vi "3-1.vi"(9 "信号数组(V)":dbl[](array[numeric]), 10 "编码位数L":dbl=8.0, 11 "量化阶Δ(V)":dbl=0.02) -> (3 "还原信号数组(V)":dbl[](array[numeric]))   [LabVIEW 2018]
panel:
  out "量化误差(V)":dbl[](array[numeric])
  out "编码数组":digitaldata
  # "输入"
  # "输出"
  # "默认编码长度L为8bit，可以自行增加变量修改\n子VI中有编码长度接口"
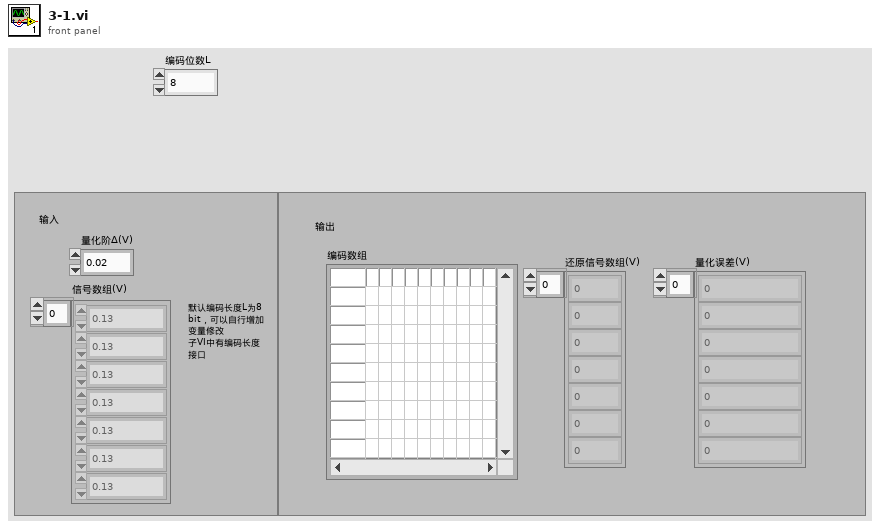
[diagram p1: front panel]
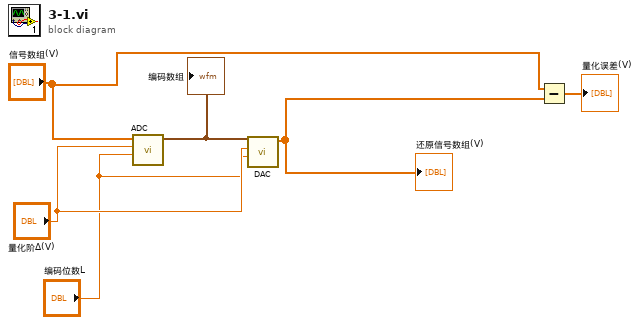
[diagram p0: block diagram]
diagram:
  n1 = call "ADC.vi"("编码位数L"="编码位数L", "量化阶Δ(V)"="量化阶Δ(V)", "信号数组(V)"="信号数组(V)") -> ("编码数组"=w6:digitaldata)  [unwired: 8 in]
  "编码数组" <- w6
  n2 = call "DAC.vi"("编码位数L"="编码位数L", "量化阶Δ(V)"="量化阶Δ(V)", "编码信号数组"=w6) -> ("还原信号数组"=w3:dbl[])  [unwired: 8 in]
  "还原信号数组(V)" <- w3
  n3 = Subtract(x="信号数组(V)", y=w3) -> (x-y=→"量化误差(V)":dbl[])
